vi "Code Hexadecimal.vi"(8 "Error In":errorcluster caption="Entrée d'erreur", 9 "Etat":bool, 10 "Numéro Relais":dbl=1.0, 11 "tableau code":u8[](array[numeric]) format="%x") -> (0 "Error Out":errorcluster caption="Sortie d'erreur", 3 "tableau en sortie":u8[](array[numeric]) format="%x")   [LabVIEW 2017]
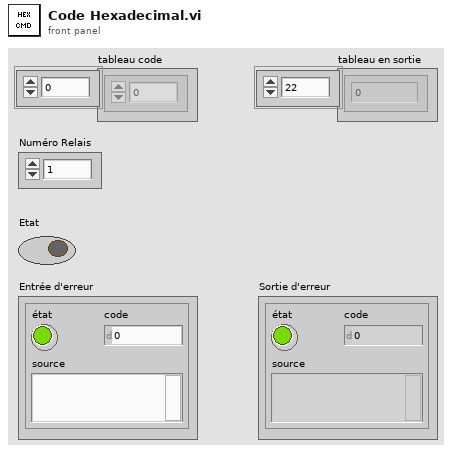
[diagram p1: front panel]
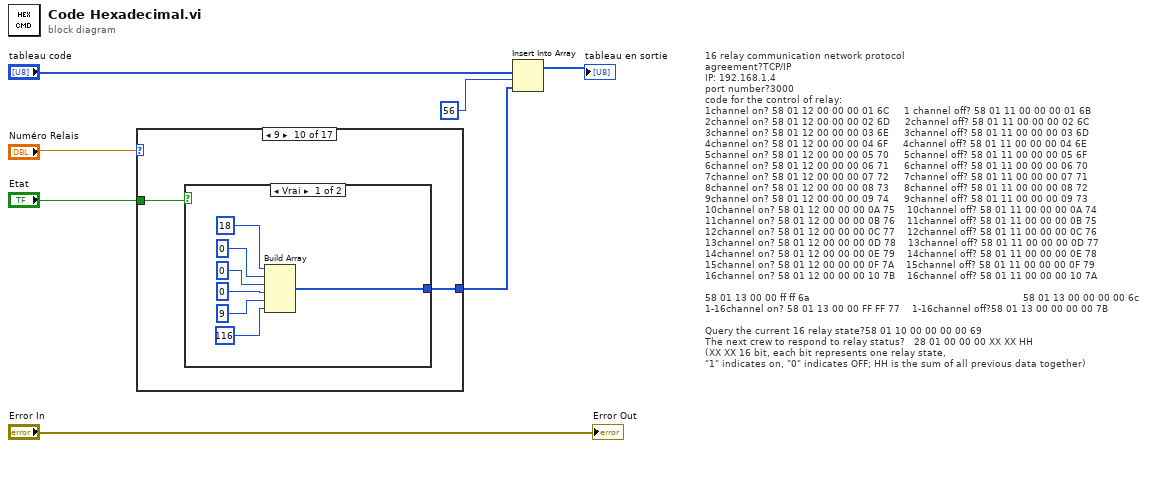
[diagram p0: block diagram]
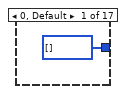
[diagram p2: hidden frame]
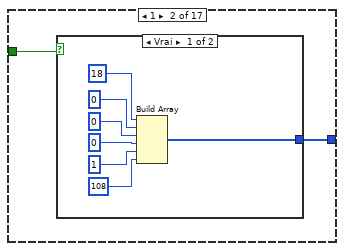
[diagram p3: hidden frame]
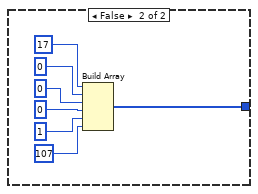
[diagram p4: hidden frame]
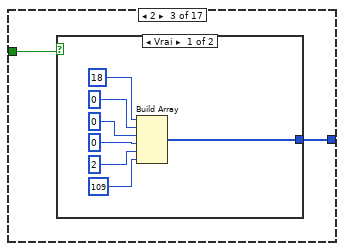
[diagram p5: hidden frame]
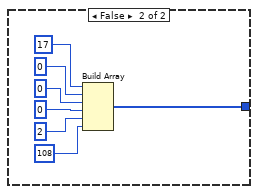
[diagram p6: hidden frame]
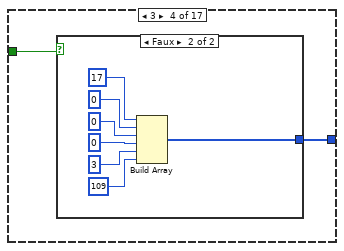
[diagram p7: hidden frame]
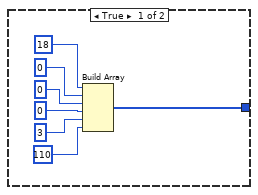
[diagram p8: hidden frame]
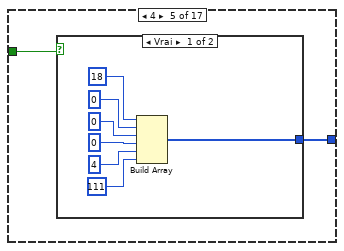
[diagram p9: hidden frame]
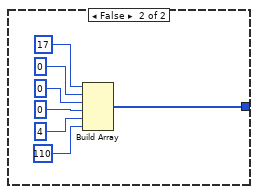
[diagram p10: hidden frame]
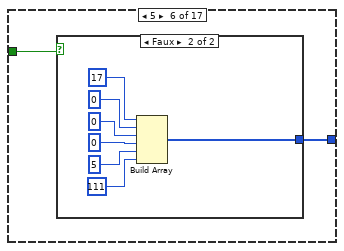
[diagram p11: hidden frame]
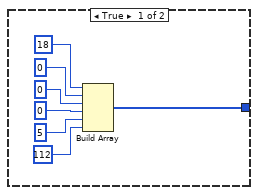
[diagram p12: hidden frame]
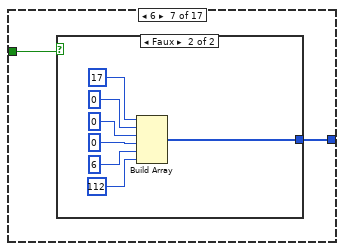
[diagram p13: hidden frame]
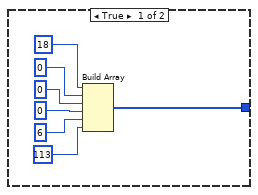
[diagram p14: hidden frame]
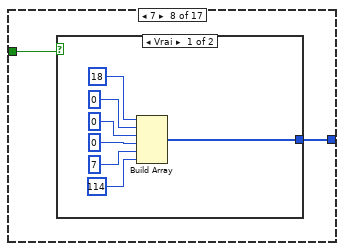
[diagram p15: hidden frame]
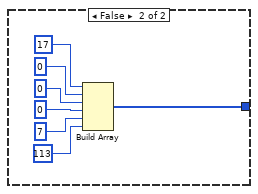
[diagram p16: hidden frame]
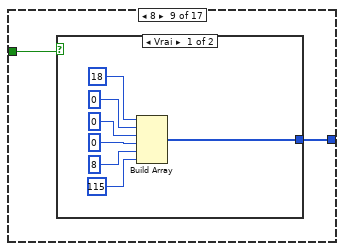
[diagram p17: hidden frame]
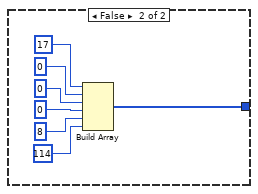
[diagram p18: hidden frame]
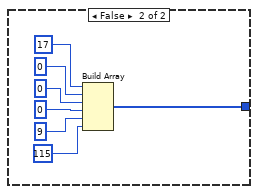
[diagram p19: hidden frame]
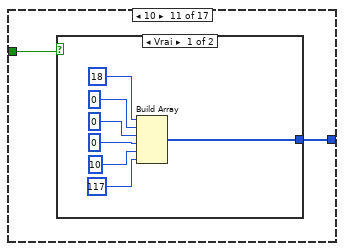
[diagram p20: hidden frame]
diagram:
  # "16 relay communication network protocol\nagreement?TCP/IP\nIP: 192.168.1.4\nport number?3000 \ncode for the control of relay:\n1channel on? 58 01 12 00 00 00 01 6C     1 channel off? 58 01 11 00 00 00 01 6B\n2channel on? 58 01 12 00 00 00 02 6D     2channel off? 58 01 11 00 00 00 02 6C\n3channel on? 58 01 12 00 00 00 03 6E     3channel off? 58 01 11 00 00 00 03 6D\n4channel on? 58 01 12 00 00 00 04 6F     4channel off? 58 01 11 00 00 00 04 6E\n5channel on? 58 01 12 00 00 00 05 70     5channel off? 58 01 11 00 00 00 05 6F\n6channel on? 58 01 12 00 00 00 06 71     6channel off? 58 01 11 00 00 00 06 70\n7channel on? 58 01 12 00 00 00 07 72     7channel off? 58 01 11 00 00 00 07 71\n8channel on? 58 01 12 00 00 00 08 73     8channel off? 58 01 11 00 00 00 08 72\n9channel on? 58 01 12 00 00 00 09 74     9channel off? 58 01 11 00 00 00 09 73\n10channel on? 58 01 12 00 00 00 0A 75    10channel off? 58 01 11 00 00 00 0A 74\n11channel on? 58 01 12 00 00 00 0B 76    11channel off? 58 01 11 00 00 00 0B 75\n12channel on? 58 01 12 00 00 00 0C 77    12channel off? 58 01 11 00 00 00 0C 76\n13channel on? 58 01 12 00 00 00 0D 78    13channel off? 58 01 11 00 00 00 0D 77\n14channel on? 58 01 12 00 00 00 0E 79    14channel off? 58 01 11 00 00 00 0E 78\n15channel on? 58 01 12 00 00 00 0F 7A    15channel off? 58 01 11 00 00 00 0F 79\n16channel on? 58 01 12 00 00 00 10 7B    16channel off? 58 01 11 00 00 00 10 7A\n\n58 01 13 00 00 ff ff 6a                                                                       58 01 13 00 00 00 00 6c\n1-16channel on? 58 01 13 00 00 FF FF 77    1-16channel off?58 01 13 00 00 00 00 7B\n\nQuery the current 16 relay state?58 01 10 00 00 00 00 69\nThe next crew to respond to relay status?   28 01 00 00 00 XX XX HH   \n(XX XX 16 bit, each bit represents one relay state, \n\"1\" indicates on, \"0\" indicates OFF; HH is the sum of all previous data together)"
  n1 = case shown="9" "Numéro Relais" {
    tunnel: "Etat" -> [_ w10 w26 w42 w58 w74 w90 w106 w122 w138 w154 w170 w186 w202 w218 w234 w250]
    tunnel: [u8[] [] w9 w25 w41 w57 w73 w89 w105 w121 w137 w153 w169 w185 w201 w217 w233 w249] -> w2
    frame 0, Default {
    }
    frame 1 {
      n2 = case shown="Vrai" w10 {
        tunnel: [w11 w18] -> w9
        frame True {
          n3 = Build Array(u8 18 ("élément"), u8 0 ("élément"), u8 0 ("élément"), u8 0 ("élément"), u8 1 ("élément"), u8 108 ("élément")) -> (w11:u8[])
        }
        frame False {
          n4 = Build Array(u8 17 ("élément"), u8 0 ("élément"), u8 0 ("élément"), u8 0 ("élément"), u8 1 ("élément"), u8 107 ("élément")) -> (w18:u8[])
        }
      }
    }
    frame 2 {
      n5 = case shown="Vrai" w26 {
        tunnel: [w27 w34] -> w25
        frame True {
          n6 = Build Array(u8 18 ("élément"), u8 0 ("élément"), u8 0 ("élément"), u8 0 ("élément"), u8 2 ("élément"), u8 109 ("élément")) -> (w27:u8[])
        }
        frame False {
          n7 = Build Array(u8 17 ("élément"), u8 0 ("élément"), u8 0 ("élément"), u8 0 ("élément"), u8 2 ("élément"), u8 108 ("élément")) -> (w34:u8[])
        }
      }
    }
    frame 3 {
      n8 = case shown="Faux" w42 {
        tunnel: [w43 w50] -> w41
        frame True {
          n9 = Build Array(u8 18 ("élément"), u8 0 ("élément"), u8 0 ("élément"), u8 0 ("élément"), u8 3 ("élément"), u8 110 ("élément")) -> (w43:u8[])
        }
        frame False {
          n10 = Build Array(u8 17 ("élément"), u8 0 ("élément"), u8 0 ("élément"), u8 0 ("élément"), u8 3 ("élément"), u8 109 ("élément")) -> (w50:u8[])
        }
      }
    }
    frame 4 {
      n11 = case shown="Vrai" w58 {
        tunnel: [w59 w66] -> w57
        frame True {
          n12 = Build Array(u8 18 ("élément"), u8 0 ("élément"), u8 0 ("élément"), u8 0 ("élément"), u8 4 ("élément"), u8 111 ("élément")) -> (w59:u8[])
        }
        frame False {
          n13 = Build Array(u8 17 ("élément"), u8 0 ("élément"), u8 0 ("élément"), u8 0 ("élément"), u8 4 ("élément"), u8 110 ("élément")) -> (w66:u8[])
        }
      }
    }
    frame 5 {
      n14 = case shown="Faux" w74 {
        tunnel: [w75 w82] -> w73
        frame True {
          n15 = Build Array(u8 18 ("élément"), u8 0 ("élément"), u8 0 ("élément"), u8 0 ("élément"), u8 5 ("élément"), u8 112 ("élément")) -> (w75:u8[])
        }
        frame False {
          n16 = Build Array(u8 17 ("élément"), u8 0 ("élément"), u8 0 ("élément"), u8 0 ("élément"), u8 5 ("élément"), u8 111 ("élément")) -> (w82:u8[])
        }
      }
    }
    frame 6 {
      n17 = case shown="Faux" w90 {
        tunnel: [w91 w98] -> w89
        frame True {
          n18 = Build Array(u8 18 ("élément"), u8 0 ("élément"), u8 0 ("élément"), u8 0 ("élément"), u8 6 ("élément"), u8 113 ("élément")) -> (w91:u8[])
        }
        frame False {
          n19 = Build Array(u8 17 ("élément"), u8 0 ("élément"), u8 0 ("élément"), u8 0 ("élément"), u8 6 ("élément"), u8 112 ("élément")) -> (w98:u8[])
        }
      }
    }
    frame 7 {
      n20 = case shown="Vrai" w106 {
        tunnel: [w107 w114] -> w105
        frame True {
          n21 = Build Array(u8 18 ("élément"), u8 0 ("élément"), u8 0 ("élément"), u8 0 ("élément"), u8 7 ("élément"), u8 114 ("élément")) -> (w107:u8[])
        }
        frame False {
          n22 = Build Array(u8 17 ("élément"), u8 0 ("élément"), u8 0 ("élément"), u8 0 ("élément"), u8 7 ("élément"), u8 113 ("élément")) -> (w114:u8[])
        }
      }
    }
    frame 8 {
      n23 = case shown="Vrai" w122 {
        tunnel: [w123 w130] -> w121
        frame True {
          n24 = Build Array(u8 18 ("élément"), u8 0 ("élément"), u8 0 ("élément"), u8 0 ("élément"), u8 8 ("élément"), u8 115 ("élément")) -> (w123:u8[])
        }
        frame False {
          n25 = Build Array(u8 17 ("élément"), u8 0 ("élément"), u8 0 ("élément"), u8 0 ("élément"), u8 8 ("élément"), u8 114 ("élément")) -> (w130:u8[])
        }
      }
    }
    frame 9 {
      n26 = case shown="Vrai" w138 {
        tunnel: [w139 w146] -> w137
        frame True {
          n27 = Build Array(u8 18 ("élément"), u8 0 ("élément"), u8 0 ("élément"), u8 0 ("élément"), u8 9 ("élément"), u8 116 ("élément")) -> (w139:u8[])
        }
        frame False {
          n28 = Build Array(u8 17 ("élément"), u8 0 ("élément"), u8 0 ("élément"), u8 0 ("élément"), u8 9 ("élément"), u8 115 ("élément")) -> (w146:u8[])
        }
      }
    }
    frame 10 {
      n29 = case shown="Vrai" w154 {
        tunnel: [w155 w162] -> w153
        frame True {
          n30 = Build Array(u8 18 ("élément"), u8 0 ("élément"), u8 0 ("élément"), u8 0 ("élément"), u8 10 ("élément"), u8 117 ("élément")) -> (w155:u8[])
        }
        frame False {
          n31 = Build Array(u8 17 ("élément"), u8 0 ("élément"), u8 0 ("élément"), u8 0 ("élément"), u8 10 ("élément"), u8 116 ("élément")) -> (w162:u8[])
        }
      }
    }
    frame 11 {
      n32 = case shown="Faux" w170 {
        tunnel: [w171 w178] -> w169
        frame True {
          n33 = Build Array(u8 18 ("élément"), u8 0 ("élément"), u8 0 ("élément"), u8 0 ("élément"), u8 11 ("élément"), u8 118 ("élément")) -> (w171:u8[])
        }
        frame False {
          n34 = Build Array(u8 17 ("élément"), u8 0 ("élément"), u8 0 ("élément"), u8 0 ("élément"), u8 11 ("élément"), u8 117 ("élément")) -> (w178:u8[])
        }
      }
    }
    frame 12 {
      n35 = case shown="Vrai" w186 {
        tunnel: [w187 w194] -> w185
        frame True {
          n36 = Build Array(u8 18 ("élément"), u8 0 ("élément"), u8 0 ("élément"), u8 0 ("élément"), u8 12 ("élément"), u8 119 ("élément")) -> (w187:u8[])
        }
        frame False {
          n37 = Build Array(u8 17 ("élément"), u8 0 ("élément"), u8 0 ("élément"), u8 0 ("élément"), u8 12 ("élément"), u8 118 ("élément")) -> (w194:u8[])
        }
      }
    }
    frame 13 {
      n38 = case shown="Faux" w202 {
        tunnel: [w203 w210] -> w201
        frame True {
          n39 = Build Array(u8 18 ("élément"), u8 0 ("élément"), u8 0 ("élément"), u8 0 ("élément"), u8 13 ("élément"), u8 120 ("élément")) -> (w203:u8[])
        }
        frame False {
          n40 = Build Array(u8 17 ("élément"), u8 0 ("élément"), u8 0 ("élément"), u8 0 ("élément"), u8 13 ("élément"), u8 119 ("élément")) -> (w210:u8[])
        }
      }
    }
    frame 14 {
      n41 = case shown="Vrai" w218 {
        tunnel: [w219 w226] -> w217
        frame True {
          n42 = Build Array(u8 18 ("élément"), u8 0 ("élément"), u8 0 ("élément"), u8 0 ("élément"), u8 14 ("élément"), u8 121 ("élément")) -> (w219:u8[])
        }
        frame False {
          n43 = Build Array(u8 17 ("élément"), u8 0 ("élément"), u8 0 ("élément"), u8 0 ("élément"), u8 14 ("élément"), u8 120 ("élément")) -> (w226:u8[])
        }
      }
    }
    frame 15 {
      n44 = case shown="Faux" w234 {
        tunnel: [w235 w242] -> w233
        frame True {
          n45 = Build Array(u8 18 ("élément"), u8 0 ("élément"), u8 0 ("élément"), u8 0 ("élément"), u8 15 ("élément"), u8 122 ("élément")) -> (w235:u8[])
        }
        frame False {
          n46 = Build Array(u8 17 ("élément"), u8 0 ("élément"), u8 0 ("élément"), u8 0 ("élément"), u8 15 ("élément"), u8 121 ("élément")) -> (w242:u8[])
        }
      }
    }
    frame 16 {
      n47 = case shown="Vrai" w250 {
        tunnel: [w251 w258] -> w249
        frame True {
          n48 = Build Array(u8 18 ("élément"), u8 0 ("élément"), u8 0 ("élément"), u8 0 ("élément"), u8 16 ("élément"), u8 123 ("élément")) -> (w251:u8[])
        }
        frame False {
          n49 = Build Array(u8 17 ("élément"), u8 0 ("élément"), u8 0 ("élément"), u8 0 ("élément"), u8 16 ("élément"), u8 122 ("élément")) -> (w258:u8[])
        }
      }
    }
  }
  n50 = Insert Into Array(array="tableau code", index=56 ("indice"), new element=w2) -> (→"tableau en sortie":u8[])
  "Error Out" <- "Error In"
